vi "1D_Jacobi_eigenvalue_algorithm_v1.vi"() -> ()   [LabVIEW 2020]
uses:
  <vilib>/Analysis/Matrix/Datatypes/RealMatrix.ctl
  <vilib>/Analysis/baseanly.llb/Real A x B.vi
  <vilib>/Analysis/baseanly.llb/Mean (DBL).vi
  <vilib>/Analysis/Matrix/Numeric/Conversions/Array To Matrix - RA2.vi
  <vilib>/Analysis/Matrix/Numeric/Conversions/Matrix To Array - RM.vi
  <vilib>/Analysis/7linalg.llb/Real Eigenvalues and Vectors.vi
  <vilib>/Analysis/Matrix/NI_Matrix.lvlib
  <vilib>/Analysis/NI_AALBase.lvlib
  <vilib>/Analysis/NI_AALPro.lvlib
panel:
  out "output array":sgl[][](array[numeric])
  out "Real Matrix":T1
  out "percent error":dbl
  out "FPGA Jacobi eigenvalue":sgl[](array[numeric])
  in  "Number of Rotations":i32=100
  out "A":dbl[][](array[numeric])
  out "LabVIEW eigvals":dbl[](array[numeric])
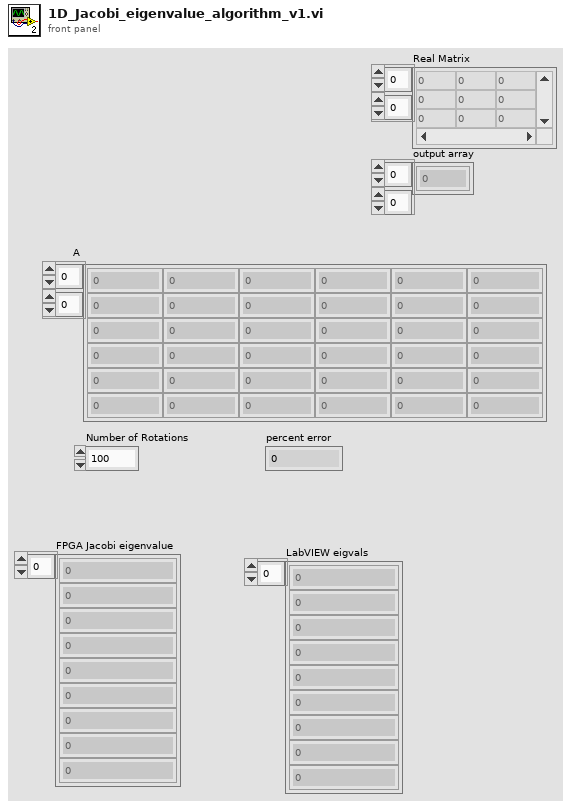
[diagram p1: front panel]
types:
  T1 = typedef "NI_Matrix.lvlib/RealMatrix.ctl" = dbl[][]
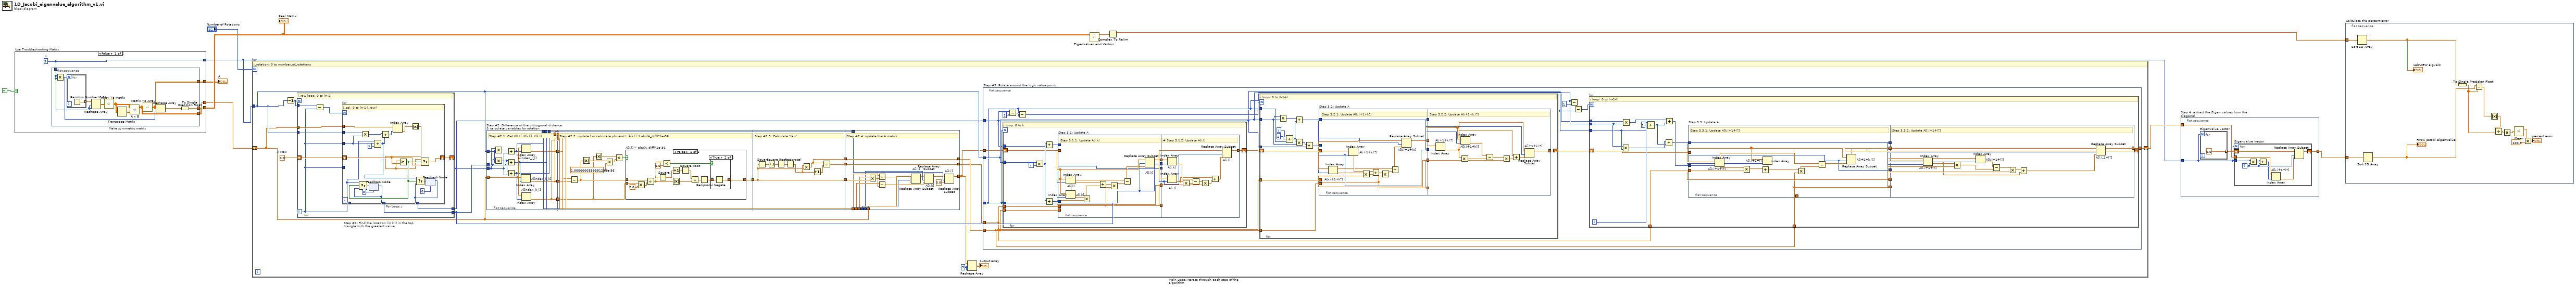
[diagram p0: block diagram]
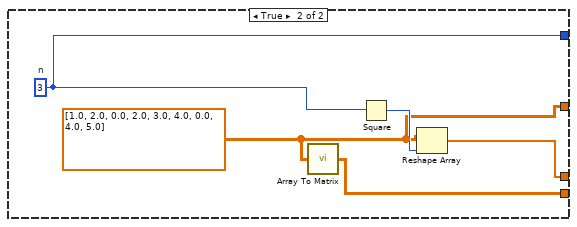
[diagram p2: hidden frame]
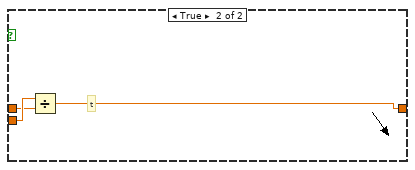
[diagram p4: hidden frame]
diagram:
  n1 = case "Use Troubleshooting Matrix" shown="False" TRUE {
    tunnel: [w13 w30] -> w9
    tunnel: [w14 w29] -> w6
    tunnel: [w12 w26] -> w3
    tunnel: [w11 w27] -> w1
    frame False {
      w11 = 3  # n
      n2 = flat-sequence "Make symmetric matrix" {
        tunnel: [w20] -> w13
        tunnel: [w18] -> w14
        tunnel: [w16] -> w12
        tunnel: w11 -> [w15]
        frame #0 {
          n3 = Multiply(x=w15, y=w15) -> (x*y=w17:i32)
          n4 = for {
            N: w17 -> [_]
            tunnel: [w25] -> w24 mode=indexing
            n5 = Random Number (0-1)() -> (number: 0 to 1=w25:dbl)
          }
          n6 = Reshape Array(w24, w15, w15) -> (w23:dbl[][])
          n7 = call-poly <vilib>:"Array To Matrix.vi"("Real 2D Array"=w23) -> ("Real Matrix"=w22:T1)
          n8 = Transpose Matrix(1:w22) -> (0:w21:T1)
          n9 = call-poly <vilib>:"A x B.vi"("B"=w21, "A"=w22) -> ("A x B"=w20:T1)  [unwired: 1 out]
          n10 = call-poly <vilib>:"Matrix To Array.vi"("Real Matrix"=w20) -> ("Real 2D Array"=w16:dbl[][])
          n11 = Reshape Array(w16, w17) -> (w19:dbl[])
          n12 = To Single Precision Float(number=w19) -> (single precision float=w18:sgl[])
        }
      }
    }
    frame True {
      w26 = sgl[][] [[1.0, 2.0, 0.0], [2.0, 3.0, 4.0], [0.0, 4.0, 5.0]]
      w27 = 3  # n
      n13 = call-poly <vilib>:"Array To Matrix.vi"("Real 2D Array"=w26) -> ("Real Matrix"=w30:T1)
      n14 = Square(x=w27) -> (x^2=w28:i32)
      n15 = Reshape Array(w26, w28) -> (w29:sgl[])
    }
  }
  "A" <- w3
  "Real Matrix" <- w9
  n16 = for "Main Loop: Iterate through each step of the algorithm" {
    N: "Number of Rotations" -> [_]
    tunnel: w1 -> [w52]
    shift-right: [w35] -> w7
    shift-left: w6 -> [w34]
    w32 = 3 ("dimension size")
    w55 = sgl 0.0  # A Max
    # "i_rotation: 0 to number_of_rotations"
    n17 = Decrement(x=w52) -> (x-1=w54:i32)
    n18 = for "Step #1: Find the location (in k,l) in the top triangle with the greatest value" {
      N: w54 -> [_]
      tunnel: w54 -> [w267]
      shift-right: [w271] -> _
      shift-left: w55 -> [w269]
      tunnel: [w270] -> w49
      tunnel: [w268] -> w53
      tunnel: w34 -> [w266]
      tunnel: w52 -> [w264]
      i -> [w265]
      # "i_row loop, 0 to (n-1)"
      n19 = Subtract(x=w267, y=w265) -> (x-y=w272:i32)
      n20 = for "For Loop: j" {
        N: w272 -> [_]
        tunnel: w265 -> [_]
        shift-right: [w290] -> w271
        shift-left: w269 -> [w291]
        tunnel: [w288] -> w270
        tunnel: [w285] -> w268
        tunnel: w265 -> [w281]
        tunnel: w266 -> [w282]
        tunnel: w265 -> [w279]
        tunnel: w264 -> [w278]
        # "j_col, 0 to (n-1-i_row)"
        n21 = Multiply(x=w278, y=w279) -> (x*y=w275:i32)
        n22 = feedback #1(0) -> (w285:i32)
        n23 = Compound Arithmetic op=unknown(w281, w279, 1 ("value")) -> (w274:i32)
        n24 = Add(x=w275, y=w274) -> (x+y=w273:i32)
        n25 = Index Array(array=w282, index=w273) -> (element=w277:sgl)
        n26 = Absolute Value(x=w277) -> (abs(x)=w276:sgl)
        n27 = Greater Or Equal?(x=w276, y=w291) -> (x >= y?=w286:bool)
        n28 = Select(t=w281, s=w286, f=w285) -> (s? t:f=w287:i32)
        n29 = feedback-in #1(w287) -> ()
        n30 = Select(t=w276, s=w286, f=w291) -> (s? t:f=w290:sgl)
        n31 = feedback #2(0) -> (w288:i32)
        n32 = Select(t=w274, s=w286, f=w288) -> (s? t:f=w289:i32)
        n33 = feedback-in #2(w289) -> ()
      }
    }
    n34 = flat-sequence "Step #2: Difference of the orthogonal distance & calculate variables for rotation" {
      tunnel: [w63] -> w48
      tunnel: [w62] -> w47
      tunnel: [w61] -> w46
      tunnel: w53 -> [w67]
      tunnel: w52 -> [w66]
      tunnel: w49 -> [w65]
      tunnel: w34 -> [w64]
      tunnel: [w63] -> w41
      tunnel: [w62] -> w40
      tunnel: [w61] -> w39
      tunnel: [w60] -> w38
      tunnel: [w59] -> w37
      tunnel: [w58] -> w36
      tunnel: [w72] -> w45
      tunnel: w48 -> [w70]
      tunnel: w47 -> [w69]
      tunnel: w46 -> [w68]
      tunnel: w45 -> [w100]
      tunnel: [w100] -> w44
      tunnel: [w99] -> w43
      tunnel: [w98] -> w42
      tunnel: [w121] -> w50
      tunnel: [w122] -> w51
      tunnel: w44 -> [w120]
      tunnel: w43 -> [w122]
      tunnel: w42 -> [w121]
      tunnel: w41 -> [w119]
      tunnel: w40 -> [w118]
      tunnel: w39 -> [w117]
      tunnel: w34 -> [w116]
      tunnel: w38 -> [w115]
      tunnel: w37 -> [w114]
      tunnel: w36 -> [w113]
      tunnel: [w112] -> w33
      frame #0 {
        # "Step #2.1: Get K[I,I], K[k,k], K[k,l]"
        n35 = Multiply(x=w65, y=w66) -> (x*y=w57:i32)
        n36 = Multiply(x=w67, y=w66) -> (x*y=w56:i32)
        n37 = Add(x=w57, y=w65) -> (x+y=w60:i32)
        n38 = Add(x=w56, y=w67) -> (x+y=w59:i32)
        n39 = Add(x=w56, y=w65) -> (x+y=w58:i32)
        n40 = Index Array "A[index_k_k]"(array=w64, index=w59) -> (element=w62:sgl)
        n41 = Index Array "A[index_k_l]"(array=w64, index=w58) -> (element=w61:sgl)
        n42 = Index Array "A[index_l_l]"(array=w64, index=w60) -> (element=w63:sgl)
      }
      frame #1 {
        # "Step #2.2: update t or calculate phi and t, A[k,l] < abs(A_diff)*1e-36"
        n43 = Subtract(x=w70, y=w69) -> (x-y=w71:sgl)
        n44 = Absolute Value(x=w71) -> (abs(x)=w75:sgl)
        n45 = Absolute Value(x=w68) -> (abs(x)=w77:sgl)
        n46 = Multiply(x=w75, y=sgl 1e-36 ("x")) -> (x*y=w76:sgl)
        n47 = Less?(x=w77, y=w76) -> (x < y?=w73:bool)
        n48 = case "A[k,l] < abs(A_diff)*1e-36" shown="False" w73 {
          tunnel: w68 -> [w91 w97]
          tunnel: w71 -> [w88 w96]
          tunnel: [w78 w95] -> w72
          frame False {
            n49 = Multiply(x=w91, y=sgl 2.0) -> (x*y=w89:sgl)
            n50 = Divide(x=w88, y=w89) -> (x/y=w82:sgl)
            n51 = Square(x=w82) -> (x^2=w86:sgl)
            n52 = Less?(x=w82, y=sgl 0.0) -> (x < y?=w80:bool)
            n53 = Increment(x=w86) -> (x+1=w85:sgl)
            n54 = Absolute Value(x=w82) -> (abs(x)=w87:sgl)
            n55 = Square Root(x=w85) -> (sqrt(x)=w84:sgl)
            n56 = Add(x=w84, y=w87) -> (x+y=w83:sgl)
            n57 = Reciprocal(x=w83) -> (1/x=w79:sgl)
            n58 = case shown="True" w80 {
              tunnel: w79 -> [w92 w94]
              tunnel: [w92 w93] -> w78
              frame False {
              }
              frame True {
                n59 = Negate(x=w94) -> (-x=w93:sgl)
              }
            }
          }
          frame True {
            # "t"
            n60 = Divide(x=w97, y=w96) -> (x/y=w95:sgl)
          }
        }
      }
      frame #2 {
        # "Step #2.3: Calculate \"tau\""
        n61 = Square(x=w100) -> (x^2=w103:sgl)
        n62 = Increment(x=w103) -> (x+1=w102:sgl)
        n63 = Square Root(x=w102) -> (sqrt(x)=w101:sgl)
        n64 = Reciprocal(x=w101) -> (1/x=w105:sgl)
        n65 = Multiply(x=w105, y=w100) -> (x*y=w99:sgl)
        n66 = Increment(x=w105) -> (x+1=w104:sgl)
        n67 = Divide(x=w99, y=w104) -> (x/y=w98:sgl)
      }
      frame #3 {
        # "Step #2.4: update the A matrix"
        n68 = Multiply(x=w117, y=w120) -> (x*y=w111:sgl)
        n69 = Add(x=w119, y=w111) -> (x+y=w108:sgl)
        n70 = Subtract(x=w118, y=w111) -> (x-y=w109:sgl)
        n71 = Replace Array Subset "A[l,l]"(array=w116, new element=w108, index=w115) -> (w107:sgl[])
        n72 = Replace Array Subset "A[k,k]"(array=w107, new element=w109, index=w114) -> (w106:sgl[])
        n73 = Replace Array Subset "A[k,l]"(array=w106, new element=sgl 0.0 ("y"), index=w113) -> (w112:sgl[])
      }
    }
    n74 = Reshape Array(w33, w32, w32) -> (→"output array":sgl[][])
    n75 = flat-sequence "Step #3: Rotate around the high value point" {
      tunnel: w53 -> [w128]
      tunnel: w33 -> [w137]
      tunnel: w52 -> [w129]
      tunnel: w51 -> [w123]
      tunnel: w50 -> [w124]
      tunnel: w49 -> [w127]
      tunnel: [w126] -> w35
      frame #0 {
        n76 = for {
          N: w128 -> [_]
          tunnel: w129 -> [w238]
          tunnel: w128 -> [w237]
          tunnel: w123 -> [w232]
          tunnel: w124 -> [w236]
          tunnel: w127 -> [w233]
          shift-right: [w224] -> w136
          shift-left: w137 -> [w231]
          i -> [w239]
          # "i loop, 0 to k"
          n77 = Multiply(x=w238, y=w239) -> (x*y=w234:i32)
          n78 = Add(x=w234, y=w233) -> (x+y=w235:i32)
          n79 = Add(x=w234, y=w237) -> (x+y=w230:i32)
          n80 = flat-sequence "Step 3.1: Update A" {
            tunnel: w236 -> [w242]
            tunnel: w235 -> [w243]
            tunnel: w232 -> [w240]
            tunnel: w231 -> [w246]
            tunnel: w230 -> [w241]
            tunnel: [w244] -> w229
            tunnel: [w243] -> w228
            tunnel: [w242] -> w227
            tunnel: [w241] -> w226
            tunnel: [w240] -> w225
            tunnel: w229 -> [w263]
            tunnel: w228 -> [w253]
            tunnel: w227 -> [w262]
            tunnel: w226 -> [w259]
            tunnel: w225 -> [w257]
            tunnel: [w252] -> w224
            frame #0 {
              # "Step 3.1.1: Update A[i,k]"
              n81 = Index Array "A[i,l]"(array=w246, index=w243) -> (element=w249:sgl)
              n82 = Index Array "A[i,k]"(array=w246, index=w241) -> (element=w251:sgl)
              n83 = Multiply(x=w251, y=w242) -> (x*y=w250:sgl)
              n84 = Add(x=w249, y=w250) -> (x+y=w248:sgl)
              n85 = Multiply(x=w248, y=w240) -> (x*y=w247:sgl)
              n86 = Subtract(x=w251, y=w247) -> (x-y=w245:sgl)
              n87 = Replace Array Subset "A[i,k]"(array=w246, new element=w245, index=w241) -> (w244:sgl[])
            }
            frame #1 {
              # "# Step 3.1.2: Update A[i,l]"
              n88 = Index Array "A[i,k]"(array=w263, index=w259) -> (element=w261:sgl)
              n89 = Index Array "A[i,l]"(array=w263, index=w253) -> (element=w255:sgl)
              n90 = Multiply(x=w255, y=w262) -> (x*y=w260:sgl)
              n91 = Subtract(x=w261, y=w260) -> (x-y=w258:sgl)
              n92 = Multiply(x=w258, y=w257) -> (x*y=w256:sgl)
              n93 = Add(x=w255, y=w256) -> (x+y=w254:sgl)
              n94 = Replace Array Subset "A[i,l]"(array=w263, new element=w254, index=w253) -> (w252:sgl[])
            }
          }
        }
        n95 = Subtract(x=w127, y=1) -> (x-y=w135:i32)
        n96 = Subtract(x=w135, y=w128) -> (x-y=w133:i32)
        n97 = for {
          N: w133 -> [_]
          shift-right: [w199] -> w125
          shift-left: w136 -> [w197]
          tunnel: w128 -> [w195]
          tunnel: w129 -> [w191]
          tunnel: w127 -> [w189]
          tunnel: w124 -> [w187]
          tunnel: w123 -> [w185]
          i -> [w194]
          # "i loop, 0 to (l-1-k)"
          n98 = Multiply(x=w195, y=w191) -> (x*y=w193:i32)
          n99 = Compound Arithmetic op=ADD(w194, 1 ("value"), w195) -> (w192:i32)
          n100 = Add(x=w193, y=w192) -> (x+y=w188:i32)
          n101 = Multiply(x=w192, y=w191) -> (x*y=w190:i32)
          n102 = Add(x=w190, y=w189) -> (x+y=w186:i32)
          n103 = flat-sequence "Step 3.2: Update A" {
            tunnel: [w211] -> w198
            tunnel: w197 -> [w210]
            tunnel: w188 -> [w201]
            tunnel: w187 -> [w202]
            tunnel: w186 -> [w203]
            tunnel: w185 -> [w200]
            tunnel: [w203] -> w184
            tunnel: [w202] -> w183
            tunnel: [w201] -> w182
            tunnel: [w200] -> w181
            tunnel: [w223] -> w199
            tunnel: w198 -> [w220]
            tunnel: w184 -> [w222]
            tunnel: w183 -> [w221]
            tunnel: w182 -> [w219]
            tunnel: w181 -> [w215]
            frame #0 {
              # "Step 3.2.1: Update A[k,i+1+k?]"
              n104 = Index Array "A[k,i+1+k?]"(array=w210, index=w201) -> (element=w206:sgl)
              n105 = Index Array "A[i+1+k,l?]"(array=w210, index=w203) -> (element=w209:sgl)
              n106 = Multiply(x=w206, y=w202) -> (x*y=w208:sgl)
              n107 = Add(x=w209, y=w208) -> (x+y=w207:sgl)
              n108 = Multiply(x=w207, y=w200) -> (x*y=w205:sgl)
              n109 = Subtract(x=w206, y=w205) -> (x-y=w204:sgl)
              n110 = Replace Array Subset "A[k,i+1+k?]"(array=w210, new element=w204, index=w201) -> (w211:sgl[])
            }
            frame #1 {
              # "Step 3.2.2: Update A[i+1+k,l?]"
              n111 = Index Array "A[i+1+k,l?]"(array=w220, index=w222) -> (element=w213:sgl)
              n112 = Multiply(x=w213, y=w221) -> (x*y=w217:sgl)
              n113 = Index Array "A[k,i+1+k?]"(array=w220, index=w219) -> (element=w218:sgl)
              n114 = Subtract(x=w218, y=w217) -> (x-y=w216:sgl)
              n115 = Multiply(x=w216, y=w215) -> (x*y=w214:sgl)
              n116 = Add(x=w213, y=w214) -> (x+y=w212:sgl)
              n117 = Replace Array Subset "A[i+1+k,l?]"(array=w220, new element=w212, index=w222) -> (w223:sgl[])
            }
          }
        }
        n118 = Subtract(x=w129, y=1) -> (x-y=w131:i32)
        n119 = Subtract(x=w131, y=w127) -> (x-y=w130:i32)
        n120 = for {
          N: w130 -> [_]
          tunnel: w129 -> [w152]
          tunnel: w128 -> [w156]
          tunnel: w127 -> [w151]
          shift-right: [w148] -> w126
          shift-left: w125 -> [w146]
          tunnel: w124 -> [w144]
          tunnel: w123 -> [w142]
          i -> [w155]
          # "i loop, 0 to (n-1-l)"
          n121 = Multiply(x=w152, y=w151) -> (x*y=w150:i32)
          n122 = Multiply(x=w156, y=w152) -> (x*y=w153:i32)
          n123 = Compound Arithmetic op=ADD(w155, 1 ("value"), w151) -> (w149:i32)
          n124 = Add(x=w150, y=w149) -> (x+y=w143:i32)
          n125 = Add(x=w153, y=w149) -> (x+y=w145:i32)
          n126 = flat-sequence "Step 3.3: Update A" {
            tunnel: [w162] -> w147
            tunnel: w146 -> [w163]
            tunnel: w145 -> [w158]
            tunnel: w144 -> [w159]
            tunnel: w143 -> [w160]
            tunnel: w142 -> [w157]
            tunnel: [w160] -> w141
            tunnel: [w159] -> w140
            tunnel: [w158] -> w139
            tunnel: [w157] -> w138
            tunnel: [w180] -> w148
            tunnel: w147 -> [w177]
            tunnel: w141 -> [w179]
            tunnel: w140 -> [w178]
            tunnel: w139 -> [w176]
            tunnel: w138 -> [w172]
            frame #0 {
              # "Step 3.3.1: Update A[k,i+1+l?]"
              n127 = Index Array "A[k,i+1+l?]"(array=w163, index=w158) -> (element=w165:sgl)
              n128 = Multiply(x=w165, y=w159) -> (x*y=w168:sgl)
              n129 = Index Array "A[l,i+1+l?]"(array=w163, index=w160) -> (element=w167:sgl)
              n130 = Add(x=w168, y=w167) -> (x+y=w166:sgl)
              n131 = Multiply(x=w166, y=w157) -> (x*y=w164:sgl)
              n132 = Subtract(x=w165, y=w164) -> (x-y=w161:sgl)
              n133 = Replace Array Subset "A[i+1+k,l?]"(array=w163, new element=w161, index=w158) -> (w162:sgl[])
            }
            frame #1 {
              # "Step 3.3.2: Update A[l,i+1+l?]"
              n134 = Index Array "A[l,i+1+l?]"(array=w177, index=w179) -> (element=w170:sgl)
              n135 = Multiply(x=w170, y=w178) -> (x*y=w174:sgl)
              n136 = Index Array "A[k,i+1+l?]"(array=w177, index=w176) -> (element=w175:sgl)
              n137 = Subtract(x=w175, y=w174) -> (x-y=w173:sgl)
              n138 = Multiply(x=w173, y=w172) -> (x*y=w171:sgl)
              n139 = Add(x=w171, y=w170) -> (x+y=w169:sgl)
              n140 = Replace Array Subset "A[l,i_1+l?]"(array=w177, new element=w169, index=w179) -> (w180:sgl[])
            }
          }
        }
      }
    }
  }
  n141 = call-poly <vilib>:"Eigenvalues and Vectors.vi"("Input Matrix"=w9) -> ("Eigenvalues"=w10:cdb[])  [unwired: 2 in, 2 out]
  n142 = Complex To Re/Im(x + iy=w10) -> (x=w4:dbl[])  [unwired: 1 out]
  n143 = flat-sequence "Step 4: extract the Eigen values from the diagonal" {
    tunnel: w7 -> [w294]
    tunnel: w1 -> [w293]
    tunnel: [w292] -> w5
    frame #0 {
      n144 = for "Eigenvalue vector" {
        N: w293 -> [_]
        tunnel: [sgl 0.0] -> w295 mode=indexing
      }
      n145 = for "Eigenvalue vector" {
        N: w293 -> [_]
        shift-right: [w302] -> w292
        shift-left: w295 -> [w303]
        tunnel: w294 -> [w301]
        tunnel: w293 -> [w300]
        i -> [w298]
        n146 = Multiply(x=w300, y=w298) -> (x*y=w299:i32)
        n147 = Add(x=w299, y=w298) -> (x+y=w297:i32)
        n148 = Index Array "A[k,i+1+l?]"(array=w301, index=w297) -> (element=w296:sgl)
        n149 = Replace Array Subset(array=w303, new element=w296, index=w298) -> (w302:sgl[])
      }
    }
  }
  n150 = flat-sequence "Calculate the percent error" {
    tunnel: w5 -> [w316]
    tunnel: w4 -> [w315]
    frame #0 {
      n151 = Sort 1D Array(array=w315) -> (sorted array=w314:dbl[])
      "LabVIEW eigvals" <- w314
      n152 = Sort 1D Array(array=w316) -> (sorted array=w313:sgl[])
      "FPGA Jacobi eigenvalue" <- w313
      n153 = To Single Precision Float(number=w314) -> (single precision float=w310:sgl[])
      n154 = Subtract(x=w313, y=w310) -> (x-y=w312:sgl[])
      n155 = Absolute Value(x=w312) -> (abs(x)=w311:sgl[])
      n156 = Divide(x=w311, y=w310) -> (x/y=w309:sgl[])
      n157 = Absolute Value(x=w309) -> (abs(x)=w308:sgl[])
      n158 = call-poly <vilib>:"Mean.vi"("X"=w308) -> ("mean"=w307:dbl)  [unwired: 1 out]
      n159 = Multiply(x=w307, y=100.0) -> (x*y=→"percent error":dbl)
    }
  }
